vi "Calibration_SubVI.vi"(8 "SamplingRate(Hz)":dbl=2000.0 format="%0.2f", 10 "LED":bool, 11 "Input (V)":dbl) -> (3 "mean":dbl format="%0.2f")   [LabVIEW 2018]
uses:
  <vilib>/DAQmx/write.llb/DAQmx Write (Analog DBL 1Chan 1Samp).vi
  <vilib>/DAQmx/read.llb/DAQmx Read (Analog 1D DBL 1Chan NSamp).vi
  <vilib>/Analysis/baseanly.llb/Mean (DBL).vi
  <vilib>/DAQmx/create/channels.llb/DAQmx Create Channel (AO-Voltage-Basic).vi
  <vilib>/DAQmx/miscellaneous.llb/DAQmx Fill In Error Info.vi
  <vilib>/DAQmx/create/channels.llb/DAQmx Create Channel (AI-Voltage-Basic).vi
  <vilib>/DAQmx/configure/timing.llb/DAQmx Timing (Sample Clock).vi
  <vilib>/Analysis/NI_AALBase.lvlib
panel:
  out "Waveform Chart":dbl[](graph)
  # "405 nm(F)"
  # "470 nm(T)"
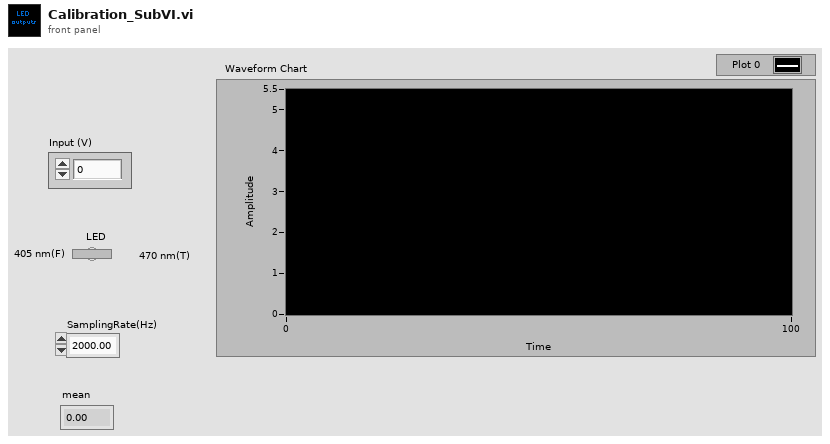
[diagram p1: front panel]
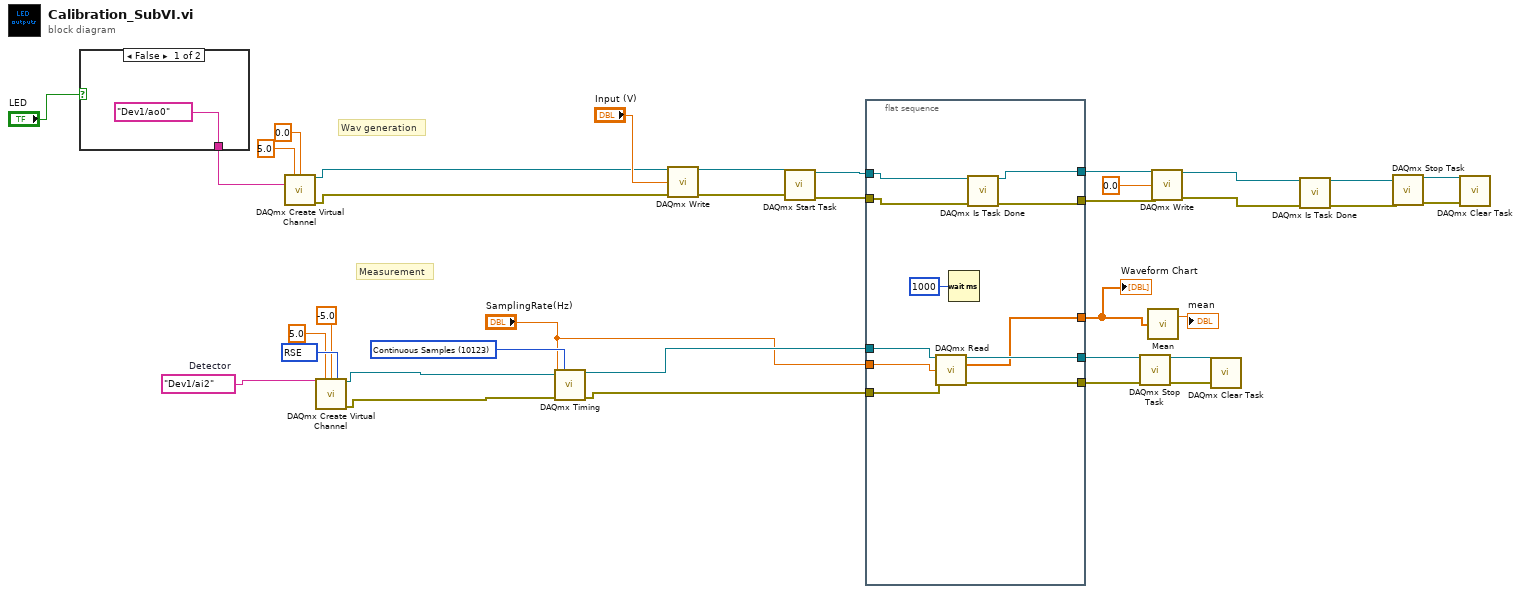
[diagram p0: block diagram]
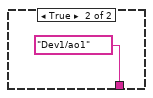
[diagram p2: hidden frame]
diagram:
  w10 = tag "Dev1/ai2"  # Detector
  w14 = 10083 items=["Default"=-1, "RSE"=10083, "NRSE"=10078, "Differential"=10106, "Pseudodifferential"=12529] ("input terminal configuration")
  w13 = 10123 items=["Finite Samples"=10178, "Continuous Samples"=10123, "Hardware Timed Single Point"=12522] ("sample mode")
  # "Measurement"
  # "Wav generation"
  n1 = case shown="False" "LED" {
    tunnel: [tag "Dev1/ao0" ("physical channels") tag "Dev1/ao1" ("physical channels")] -> w33
    frame False {
    }
    frame True {
    }
  }
  n2 = call-poly <vilib>:"DAQmx Create Virtual Channel.vi"("maximum value"=5.0, "minimum value"=0.0, "physical channels"=w33) -> ("task out"=w25:refnum<k21>, "error out"=w24:errorcluster)  [unwired: 11 in]
  n3 = call-poly <vilib>:"DAQmx Create Virtual Channel.vi"("maximum value"=5.0, "minimum value"=-5.0, "input terminal configuration"=w14, "physical channels"=w10) -> ("task out"=w15:refnum<k21>, "error out"=w16:errorcluster)  [unwired: 10 in]
  n4 = call-poly <vilib>:"DAQmx Timing.vi"("task/channels in"=w15, "sample mode"=w13, "rate"="SamplingRate(Hz)", "error in"=w16) -> ("task out"=w9:refnum<k21>, "error out"=w8:errorcluster)  [unwired: 10 in]
  n5 = call-poly <vilib>:"DAQmx Write.vi"("task/channels in"=w25, "data"="Input (V)", "error in"=w24) -> ("task out"=w28:refnum<k21>, "error out"=w29:errorcluster)  [unwired: 10 in, 1 out]
  n6 = call <vilib>:"DAQmx Start Task.vi"("task/channels in"=w28, "error in"=w29) -> ("task out"=w27:refnum<k21>, "error out"=w26:errorcluster)  [unwired: 12 in]
  n7 = flat-sequence {
    tunnel: [w45] -> w23
    tunnel: w27 -> [w48]
    tunnel: [w46] -> w22
    tunnel: w26 -> [w47]
    tunnel: w9 -> [w44]
    tunnel: w8 -> [w43]
    tunnel: [w42] -> w7
    tunnel: [w41] -> w6
    tunnel: [w40] -> w2
    tunnel: "SamplingRate(Hz)" -> [w39]
    frame #0 {
      n8 = call-poly <vilib>:"DAQmx Read.vi"("task/channels in"=w44, "number of samples per channel"=w39, "error in"=w43) -> ("task out"=w42:refnum<k21>, "data"=w40:dbl[], "error out"=w41:errorcluster)  [unwired: 10 in]
      n9 = Wait (ms)(milliseconds to wait=u32 1000) -> ()  [unwired: 1 out]
      n10 = call <vilib>:"DAQmx Is Task Done.vi"("task/channels in"=w48, "error in"=w47) -> ("task out"=w45:refnum<k21>, "error out"=w46:errorcluster)  [unwired: 11 in, 1 out]
    }
  }
  n11 = call <vilib>:"DAQmx Stop Task.vi"("task/channels in"=w7, "error in"=w6) -> ("task out"=w4:refnum<k21>, "error out"=w5:errorcluster)  [unwired: 12 in]
  n12 = call-poly <vilib>:"Mean.vi"("X"=w2) -> ("mean"=→"mean":dbl)  [unwired: 1 out]
  n13 = call-poly <vilib>:"DAQmx Write.vi"("task/channels in"=w23, "data"=0.0, "error in"=w22) -> ("task out"=w18:refnum<k21>, "error out"=w17:errorcluster)  [unwired: 10 in, 1 out]
  n14 = call <vilib>:"DAQmx Clear Task.vi"("task in"=w4, "error in"=w5) -> ()  [unwired: 13 in, 1 out]
  n15 = call <vilib>:"DAQmx Is Task Done.vi"("task/channels in"=w18, "error in"=w17) -> ("task out"=w20:refnum<k21>, "error out"=w19:errorcluster)  [unwired: 11 in, 1 out]
  n16 = call <vilib>:"DAQmx Stop Task.vi"("task/channels in"=w20, "error in"=w19) -> ("task out"=w30:refnum<k21>, "error out"=w31:errorcluster)  [unwired: 12 in]
  n17 = call <vilib>:"DAQmx Clear Task.vi"("task in"=w30, "error in"=w31) -> ()  [unwired: 13 in, 1 out]
  "Waveform Chart" <- w2
